vi "Initialize RS485.vi"(8 "error in (no error)":errorcluster, 10 "Internal?":bool, 11 "Huber Unistat 410 Settings":T1 {"Address" min=0 max=99 format="%02.0f"}) -> (0 "error out":errorcluster, 2 "Connection Error":bool, 3 "Huber Unistat 410 Settings 2":T1 {"Address" min=0 max=99})   [LabVIEW 2018, in "Huber Unistat 410 TCU.lvlib"]
uses:
  Huber Unistat 410 TCU.lvlib
  Huber Unistat 410 RS485 Settings.ctl
  <vilib>/Instr/_visa.llb/VISA Configure Serial Port (Instr).vi
  <vilib>/regexp/Match Regular Expression.xnode
panel:
  out "read string":string
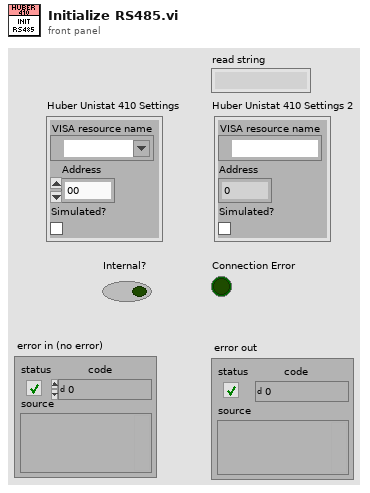
[diagram p1: front panel]
types:
  T1 = typedef "Huber Unistat 410 TCU.lvlib/Huber Unistat 410 RS485 Settings.ctl" = cluster{"VISA resource name":refnum<visa-resource-name>, "Address":i8, "Simulated?":bool}
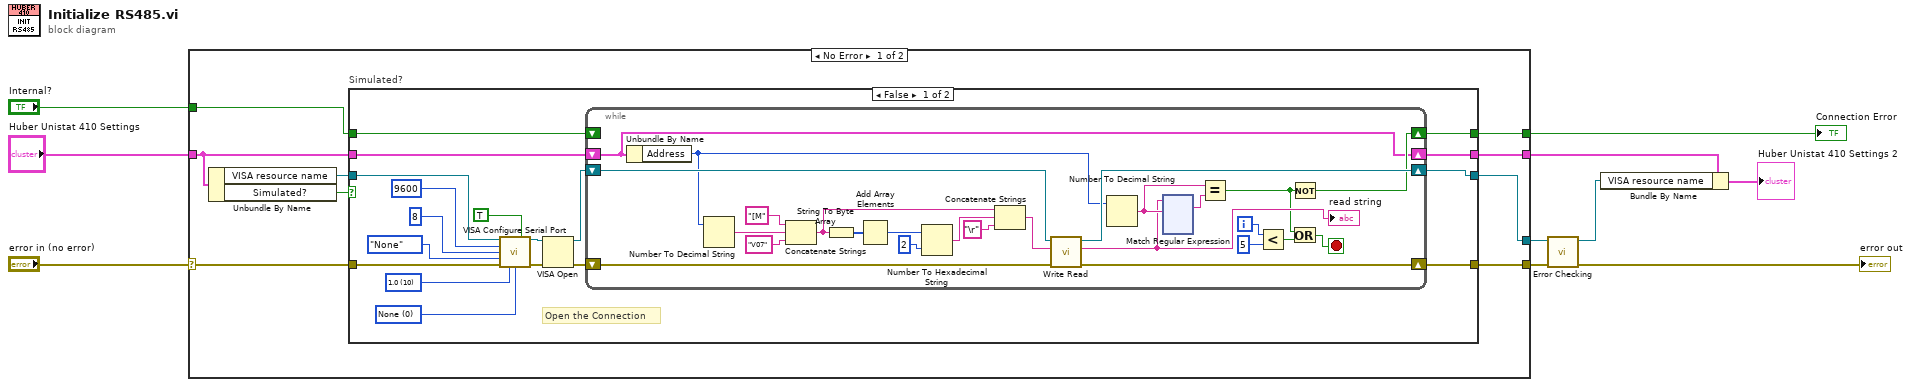
[diagram p0: block diagram]
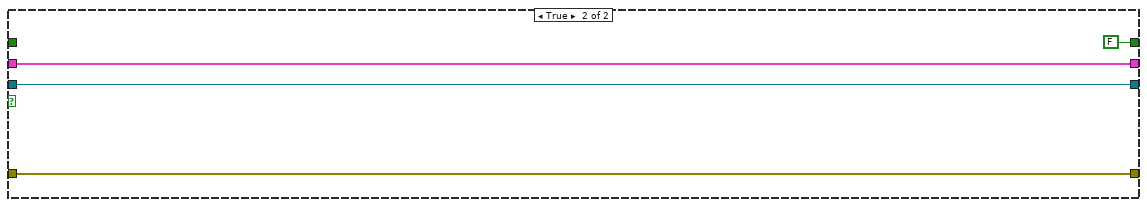
[diagram p2: hidden frame]
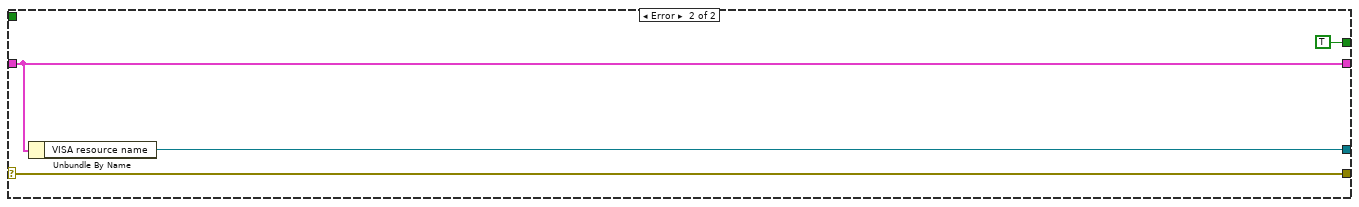
[diagram p3: hidden frame]
diagram:
  n1 = case shown="No Error" "error in (no error)" {
    selector: "error in (no error)" -> [w19 w184]
    tunnel: "Huber Unistat 410 Settings" -> [w13 w181]
    tunnel: [w18 w184] -> w8
    tunnel: [w16 w183] -> w9
    tunnel: [w14 TRUE] -> w5
    tunnel: [w12 w181] -> w4
    tunnel: "Internal?" -> [w11 _]
    frame No Error {
      n2 = Unbundle By Name(w13) -> ("VISA resource name"=w17:refnum<visa-resource-name>, "Simulated?"=w15:bool)
      n3 = case "Simulated?" shown="False" w15 {
        tunnel: w19 -> [w32 w180]
        tunnel: [w26 w180] -> w18
        tunnel: [w20 w179] -> w16
        tunnel: w17 -> [w31 w179]
        tunnel: [w28 FALSE] -> w14
        tunnel: w13 -> [w29 w177]
        tunnel: [w27 w177] -> w12
        tunnel: w11 -> [w25 _]
        frame False {
          w33 = u16 0 items=["None", "XON/XOFF", "RTS/CTS", "XON/XOFF & RTS/CTS", "DTR/DSR", "XON/XOFF & DTR/DSR"] ("flow control (0:none)")
          w34 = u16 10 items=["1.0"=10, "1.5"=15, "2.0"=20] ("stop bits (10: 1 bit)")
          # "Open the Connection"
          n4 = call-poly "VISA Configure Serial Port"("VISA resource name"=w31, "Enable Termination\nChar (T)"=TRUE ("Enable Termination\nChar (T)"), "baud rate (9600)"=u32 9600, "data bits (8)"=u16 8, "parity (0:none)"=enum16{"None", "Odd", "Even", "Mark", "Space"}."None", "error in (no error)"=w32, "stop bits (10: 1 bit)"=w34, "flow control (0:none)"=w33) -> ("VISA resource name out"=w23:refnum<visa-resource-name>, "error out"=w24:errorcluster)  [unwired: 6 in]
          n5 = VISA Open(error in (no error)=w24, VISA resource name=w23) -> (VISA resource name=w21:refnum<visa-resource-name>, error out=w22:errorcluster)  [unwired: 3 in]
          n6 = while {
            shift-right: [w48] -> w26
            shift-left: w22 -> [w58]
            shift-right: [w56] -> w20
            shift-left: w21 -> [w57]
            shift-right: [w45] -> w27
            shift-left: w29 -> [w45]
            shift-right: [w46] -> w28
            shift-left: w25 -> [_]
            i -> [w62]
            stop <- w59 stop-if-true
            n7 = Unbundle By Name(w45) -> ("Address"=w49:i8)
            n8 = Number To Decimal String(number=w49) -> (decimal integer string=w53:string)  [unwired: 1 in]
            n9 = Concatenate Strings("[M" ("string"), w53, "V07" ("string")) -> (w40:string)
            n10 = String To Byte Array(string=w40) -> (unsigned byte array=w43:u8[])
            n11 = Add Array Elements(numeric array=w43) -> (sum=w44:u8)
            n12 = Number To Hexadecimal String(1:i16 2 ("width (-)"), 2:w44) -> (0:w39:string)
            n13 = Concatenate Strings(w40, w39, "\r" ("string")) -> (w38:string)
            n14 = call "Write Read.vi"("error in (no error)"=w58, "write string"=w38, "VISA Refnum in"=w57) -> ("error out"=w48:errorcluster, "read string"=w50:string, "VISA Refnum out"=w56:refnum<visa-resource-name>)  [unwired: 6 in]
            "read string" <- w50
            n15 = Number To Decimal String(number=w49) -> (decimal integer string=w52:string)  [unwired: 1 in]
            n16 = xnode "Match Regular Expression"("input string"=w50, "regular expression"=w52) -> ("whole match"=w51:string)  [unwired: 4 in, 4 out]
            n17 = Equal?(x=w52, y=w51) -> (x = y?=w47:bool)
            n18 = Less?(x=w62, y=5) -> (x < y?=w60:bool)
            n19 = Not(x=w47) -> (.not. x?=w46:bool)
            n20 = Or(x=w47, y=w60) -> (x .or. y?=w59:bool)
          }
        }
        frame True {
        }
      }
    }
    frame Error {
      n21 = Unbundle By Name(w181) -> ("VISA resource name"=w183:refnum<visa-resource-name>)
    }
  }
  "Connection Error" <- w5
  n22 = call "Error Checking.vi"("error in (no error)"=w8, "VISA resource name"=w9) -> ("error out"=→"error out":errorcluster, "VISA resource name"=w6:refnum<visa-resource-name>)  [unwired: 7 in, 1 out]
  n23 = Bundle By Name(cluster=w4, "VISA resource name"=w6) -> (→"Huber Unistat 410 Settings 2":T1)
